vi "Write Multiple Sections.vi"(7 "error in (no error)":errorcluster, 8 "Section Cluster":variant, 10 "JSON Sections":string="{}") -> (0 "error out":errorcluster, 3 "<JSON>":string caption="<JSON>Sections")   [LabVIEW 2019, in "JSONtext.lvlib"]
doc: "Merges a Cluster of Section Clusters (subclusters) into JSON Object. A \"Section Cluster\" is defined in analogy to the OpenG Variant Config Library \"Section Cluster\" functions, using a JSON Object, with subObjects representing \"Sections\", instead of INI format.\n\nMerging means that each element of the Section Cluster is inserted into the JSON \"Section\" (Object Item), using the data name of the cluster element. If a Path to the Section is not specified then the data name of the cluster is used. The Section is created if it does not exist.\n\nFor example, Merging the Cluster \"Settings\" with elements A=123 and B=\"test\" into {\"C\":2,\"Settings\":{\"A\"=6,\"D\":9}} would result in:\n{\"C\":2,\"Settings\":{\"A\"=123,\"D\":9,\"B\":\"test\"}}\n\nNote that this merging is not recursive into subClusters."
uses:
  JSONtext.lvlib
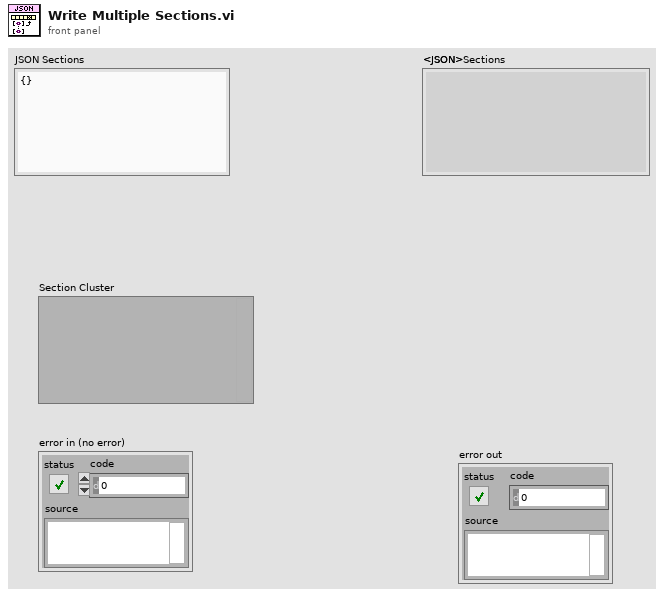
[diagram p1: front panel]
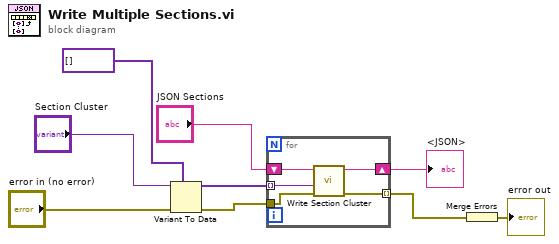
[diagram p0: block diagram]
diagram:
  n1 = Variant To Data(error in="error in (no error)", type=variant[] [], Variant="Section Cluster") -> (data=w8:variant[], error out=w2:errorcluster)
  n2 = for {
    tunnel: w8 -> [w14] mode=indexing
    shift-right: [w12] -> w4
    shift-left: "JSON Sections" -> [w13]
    tunnel: [w11] -> w3 mode=indexing
    tunnel: w2 -> [w10]
    n3 = call "Write Section Cluster.vi"("error in (no error)"=w10, "Section Cluster"=w14, "JSON Sections"=w13) -> ("error out"=w11:errorcluster, "<JSON>"=w12:string)  [unwired: 6 in]
  }
  "<JSON>" <- w4
  n4 = Merge Errors(w3) -> (→"error out":errorcluster)
